vi "Get Cluster Elements Names.vi"(8 "错误输入":errorcluster, 10 "Cluster":variant) -> (0 "错误输出":errorcluster, 2 "Elements Names":string[](array[string]))   [LabVIEW 2012, in "TD Tools.lvlib"]
uses:
  TD Tools.lvlib
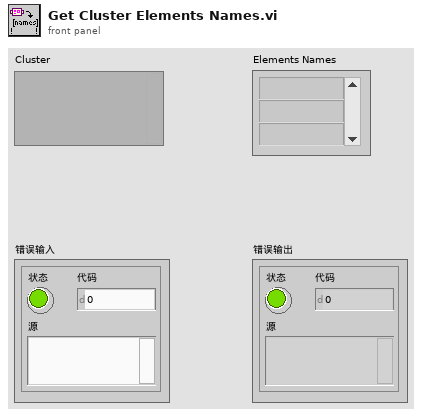
[diagram p1: front panel]
types:
  T1 = typedef "TD Tools.lvlib/Type Descriptor.ctl" = u16[]
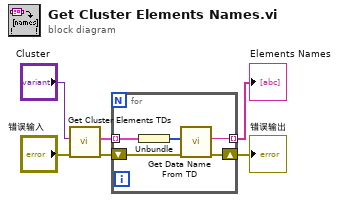
[diagram p0: block diagram]
diagram:
  n1 = call "Get Cluster Elements TDs.vi"("错误输入"="错误输入", "Cluster"="Cluster") -> ("错误输出"=w3:errorcluster, "Type Descriptors"=w4:cluster{T1}[])  [unwired: 8 in]
  n2 = for {
    tunnel: w4 -> [w11] mode=indexing
    shift-right: [w9] -> w2
    shift-left: w3 -> [w10]
    tunnel: [w7] -> w1 mode=indexing
    n3 = Unbundle(w11) -> (w8:T1)
    n4 = call "Get Data Name From TD.vi"("错误输入"=w10, "Type Descriptor"=w8) -> ("错误输出"=w9:errorcluster, "Name"=w7:string)  [unwired: 8 in]
  }
  "Elements Names" <- w1
  "错误输出" <- w2
